vi "DAQinit(allmethods).vi"(8 "error in":errorcluster, 11 "Parameters":T1) -> (0 "error out":errorcluster, 3 "INITout":refnum<class "RADEBase.lvclass">)   [LabVIEW 2014]
uses:
  <userlib>/_RADE/RIO/RADEBase/classes/RADEBase/RADEBase.lvclass
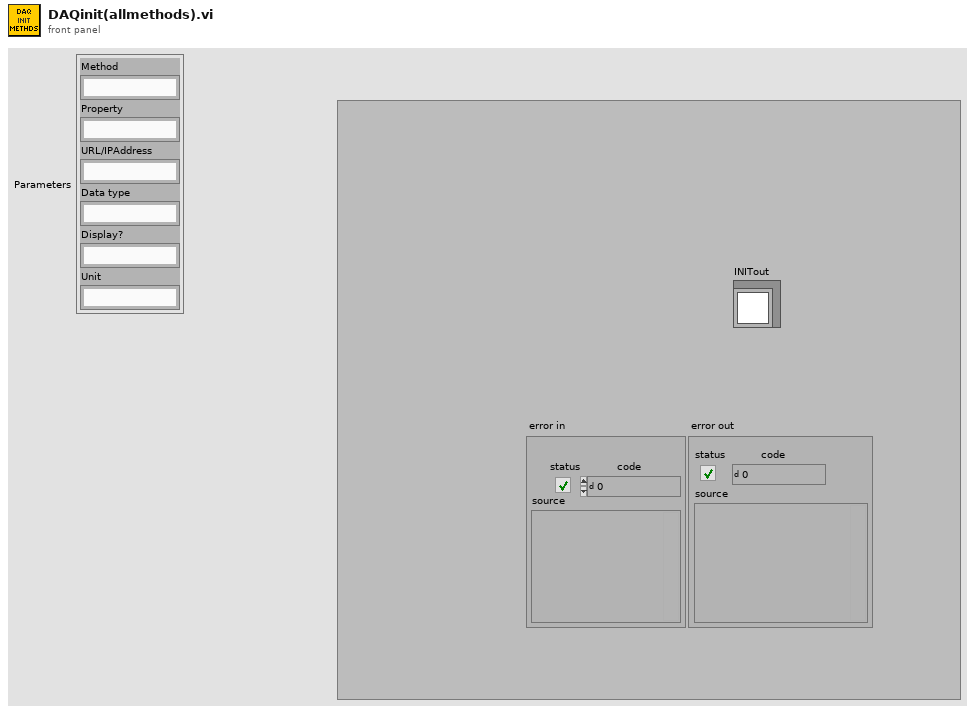
[diagram p1: front panel]
types:
  T1 = cluster{"Method":string, "Property":string, "URL/IPAddress":string, "Data type":string, "Display?":string, "Unit":string}
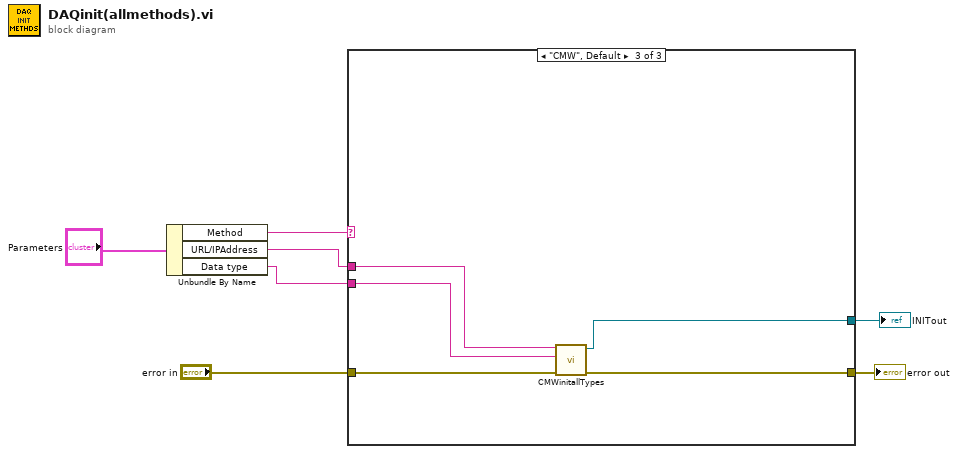
[diagram p0: block diagram]
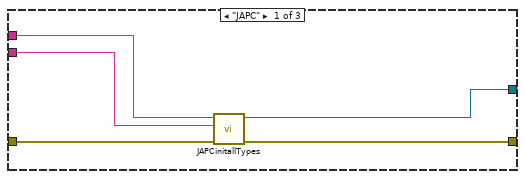
[diagram p2: hidden frame]
diagram:
  n1 = Unbundle By Name("Parameters") -> ("Method"=w2:string, "URL/IPAddress"=w5:string, "Data type"=w4:string)
  n2 = case shown="\"CMW\", Default" w2 {
    tunnel: "error in" -> [w11 w13 w17]
    tunnel: [w12 w13 w18] -> w6
    tunnel: w5 -> [w10 _ w14]
    tunnel: w4 -> [w9 _ w16]
    tunnel: [w8 _ w15] -> w3
    frame "JAPC" {
      n3 = call "JAPCinitallTypes.vi"("error in"=w11, "Data Type"=w9, "URL"=w10) -> ("error out"=w12:errorcluster, "JAPC out"=w8:refnum<class "JSubscribe.lvclass">)  [unwired: 7 in]
    }
    frame "PLC" {
      # "Since the PLC needs not be initalized, \na DEFAULT object which will not be used is passed so as to still\nhave the same index number in the parameter array"
    }
    frame "CMW", Default {
      n4 = call "CMWinitallTypes.vi"("error in"=w17, "Data Type"=w16, "URL"=w14) -> ("error out"=w18:errorcluster, "CMWout"=w15:refnum<class "CMWSubscribe.lvclass">)  [unwired: 7 in]
    }
  }
  "error out" <- w6
  "INITout" <- w3
